vi "Write Available motors.vi"(8 "error in (no error)":errorcluster, 10 "Available motors":refnum<class "Motor.lvclass">[](array[class]), 11 "Available motors in":refnum<class "Motor-assembly.lvclass">) -> (0 "error out":errorcluster, 3 "Available motors out":refnum<class "Motor-assembly.lvclass">)   [LabVIEW 2013, in "PowderDeposition.lvlib" / "Motor-assembly.lvclass"]
uses:
  Motor-assembly.lvclass
  Motor/Motor.lvclass
  Motor-assembly.lvclass/Motor-assembly.ctl
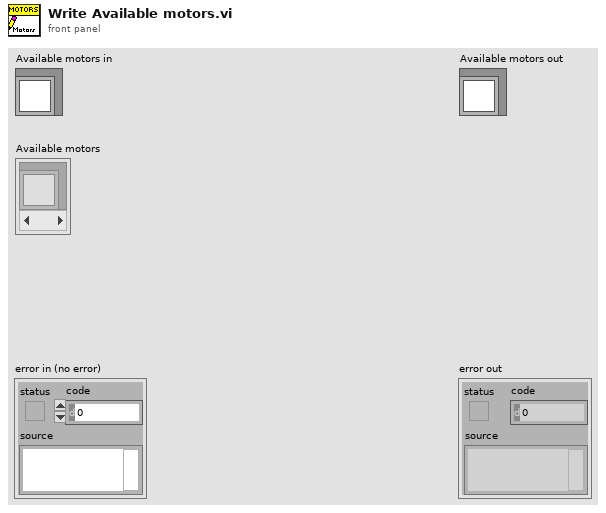
[diagram p1: front panel]
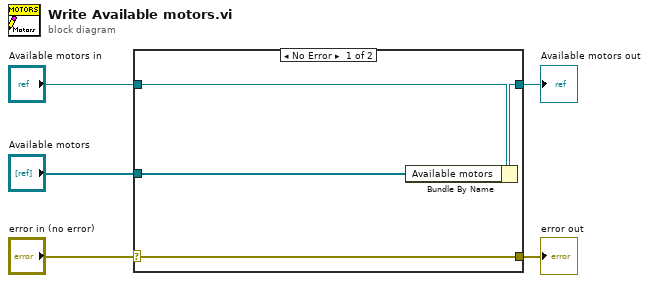
[diagram p0: block diagram]
diagram:
  n1 = case shown="No Error" "error in (no error)" {
    selector: "error in (no error)" -> [w9 w10]
    tunnel: [w9 w10] -> w4
    tunnel: [w7 w11] -> w2
    tunnel: "Available motors in" -> [w8 w11]
    tunnel: "Available motors" -> [w6 _]
    frame No Error {
      n2 = Bundle By Name(cluster=w8, "Available motors"=w6) -> (w7:refnum<class "Motor-assembly.lvclass">)
    }
    frame Error {
    }
  }
  "error out" <- w4
  "Available motors out" <- w2
